vi "Read Attributes.vi"(8 "error in (no error)":errorcluster, 11 "Element in":refnum<class "Element.lvclass">) -> (0 "error out":errorcluster, 2 "Attributes":T1[](array[typedef]), 3 "Element out":refnum<class "Element.lvclass">)   [LabVIEW 2014, in "Element.lvclass"]
uses:
  Element.lvclass
  Controls/Attribute.ctl
  Element.lvclass/Element.ctl
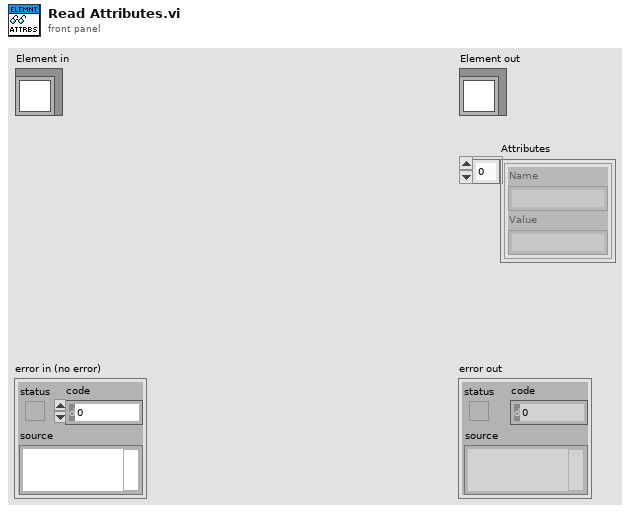
[diagram p1: front panel]
types:
  T1 = typedef "Attribute.ctl" = cluster{"Name":string, "Value":string}
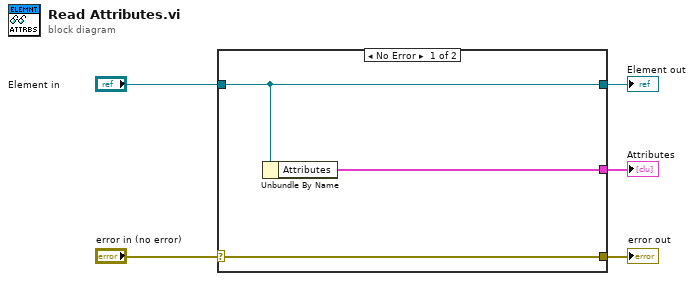
[diagram p0: block diagram]
diagram:
  n1 = case shown="No Error" "error in (no error)" {
    selector: "error in (no error)" -> [w8 w9]
    tunnel: [w8 w9] -> w4
    tunnel: [w7 w10] -> w2
    tunnel: "Element in" -> [w7 w10]
    tunnel: [w6 _] -> w1
    frame No Error {
      n2 = Unbundle By Name(w7) -> ("Attributes"=w6:T1[])
    }
    frame Error {
    }
  }
  "error out" <- w4
  "Element out" <- w2
  "Attributes" <- w1
